vi "myRIO_BRig_RT__Case_Exp_State_initTrial__CueType.vi"(4 "input_dataBlock":u16[][](array[numeric]), 6 "input_idxDataBlock_T2R":i32, 8 "input_idxDataBlock":u16, 9 "input_I_reward":bool, 10 "input_iTrial":u16, 11 "input_dataExp":u16[](array[numeric])) -> (3 "output_LED":bool)   [LabVIEW 2014]
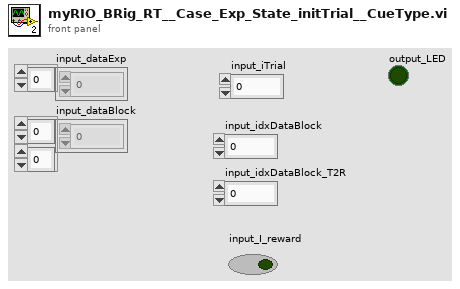
[diagram p1: front panel]
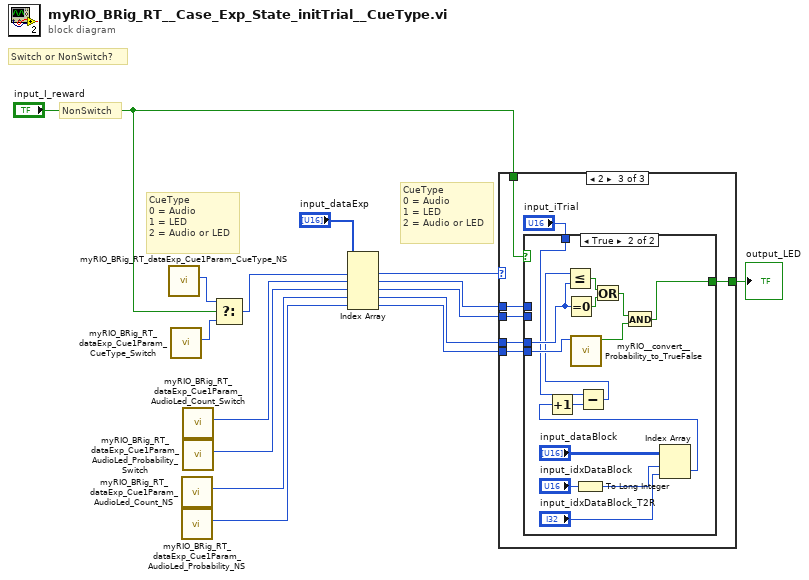
[diagram p0: block diagram]
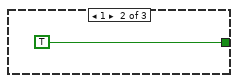
[diagram p3: hidden frame]
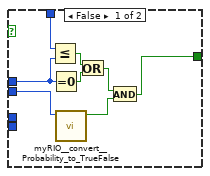
[diagram p4: hidden frame]
diagram:
  # "CueType\n0 = Audio\n1 = LED\n2 = Audio or LED"
  # "CueType\n0 = Audio\n1 = LED\n2 = Audio or LED"
  # "NonSwitch"
  # "Switch or NonSwitch?"
  n1 = call "myRIO_BRig_RT_dataExp_Cue1Param_CueType_NS.vi"() -> ("output_Cue1Param_CueType_NS"=w15:i32)  [unwired: 11 in]
  n2 = call "myRIO_BRig_RT_dataExp_Cue1Param_CueType_Switch.vi"() -> ("output_Cue1Param_CueType_Switch"=w14:i32)  [unwired: 11 in]
  n3 = call "myRIO_BRig_RT_dataExp_Cue1Param_AudioLed_Count_NS.vi"() -> ("output_Cue1Param_AudioLed_Count_NS"=w9:i32)  [unwired: 11 in]
  n4 = call "myRIO_BRig_RT_dataExp_Cue1Param_AudioLed_Probability_NS.vi"() -> ("output_Cue1Param_AudioLed_Probability_NS"=w8:i32)  [unwired: 11 in]
  n5 = call "myRIO_BRig_RT_dataExp_Cue1Param_AudioLed_Count_Switch.vi"() -> ("output_Cue1Param_AudioLed_Count_Switch"=w11:i32)  [unwired: 11 in]
  n6 = call "myRIO_BRig_RT_dataExp_Cue1Param_AudioLed_Probability_Switch.vi"() -> ("output_Cue1Param_AudioLed_Probability_Switch"=w10:i32)  [unwired: 11 in]
  n7 = Select(t=w15, s="input_I_reward", f=w14) -> (s? t:f=w12:i32)
  n8 = Index Array(array="input_dataExp", index #1=w12, index #2=w11, index #3=w10, index #4=w9, index #5=w8) -> (element #1=w7:u16, element #2=w4:u16, element #3=w3:u16, element #4=w2:u16, element #5=w1:u16)
  n9 = case shown="2" w7 {
    tunnel: [_ TRUE w17] -> w6
    tunnel: "input_I_reward" -> [_ _ w23]
    tunnel: w4 -> [_ _ w22]
    tunnel: w3 -> [_ _ w21]
    tunnel: w2 -> [_ _ w20]
    tunnel: w1 -> [_ _ w19]
    frame 0, Default {
    }
    frame 1 {
    }
    frame 2 {
      n10 = case shown="True" w23 {
        tunnel: w22 -> [w31 _]
        tunnel: w21 -> [w27 _]
        tunnel: w20 -> [_ w40]
        tunnel: w19 -> [_ w41]
        tunnel: "input_iTrial" -> [w30 w34]
        tunnel: [w24 w42] -> w17
        frame False {
          n11 = Less Or Equal?(x=w30, y=w31) -> (x <= y?=w28:bool)
          n12 = Equal To 0?(x=w31) -> (x = 0?=w29:bool)
          n13 = call "myRIO__convert__Probability_to_TrueFalse.vi"("input_probability_u16"=w27) -> ("output_TF"=w25:bool)  [unwired: 10 in]
          n14 = Or(x=w28, y=w29) -> (x .or. y?=w26:bool)
          n15 = And(x=w26, y=w25) -> (x .and. y?=w24:bool)
        }
        frame True {
          n16 = Equal To 0?(x=w40) -> (x = 0?=w46:bool)
          n17 = call "myRIO__convert__Probability_to_TrueFalse.vi"("input_probability_u16"=w41) -> ("output_TF"=w43:bool)  [unwired: 10 in]
          n18 = To Long Integer(number="input_idxDataBlock") -> (32bit integer=w37:i32)
          n19 = Index Array(array="input_dataBlock", index (row)=w37, index (col)="input_idxDataBlock_T2R") -> (element=w36:u16)
          n20 = Increment(x=w36) -> (x+1=w35:u16)
          n21 = Subtract(x=w34, y=w35) -> (x-y=w33:u16)
          n22 = Less Or Equal?(x=w33, y=w40) -> (x <= y?=w45:bool)
          n23 = Or(x=w45, y=w46) -> (x .or. y?=w44:bool)
          n24 = And(x=w44, y=w43) -> (x .and. y?=w42:bool)
        }
      }
    }
  }
  "output_LED" <- w6
